vi "AlGaInPAs_v20.vi"(2 "Debug Mode":bool, 3 "Elapsed Time(s)":dbl, 4 "State":enum16{"Edit", "Start", "Run", "End", "Idle"}(ring), 5 "Argument List In":string[](array[string])) -> (0 "Status Out":string, 1 "Argument List Out":string[](array[string]))   [LabVIEW 2011]
uses:
  high_level_proc/source_noDilute.ctl
  high_level_proc/source_noDilution.ctl
panel:
  in  "Array":refnum<vi>[](array[refnum])
  in  "Al bubbler":T1 caption="Al" {"Flow" format="%.2f"}
  in  "Se bubbler":T2={"Dilution"=FALSE, "Calculated"=0, "MFC1 flow"=0.0, "MFC2 flow"=10.0, "MFC3 flow"=100.0, "Bubbler (main)"={"Flow"=0.0, "Prep"=FALSE, "Run"=FALSE, "Active"=FALSE}} caption="Al" {"Bubbler (main)"."Flow" format="%.2f"; "MFC1 flow" format="%.4f"; "MFC3 flow" format="%.1f"; "MFC2 flow" format="%.2f"; "Calculated" items=["Flow", "MFC1", "MFC2", "MFC3"]}
  in  "P bubbler":T1 caption="Al" {"Flow" format="%.2f"}
  in  "As gas":T1 caption="Al" {"Flow" format="%.2f"}
  in  "P gas":T1 caption="Al" {"Flow" format="%.2f"}
  in  "In bubbler":T1 caption="Al" {"Flow" format="%.2f"}
  in  "Tab Control":T3(tab)
  out "Al Prep":bool caption="Pre-run"
  out "Al Run":bool caption="Run"
  out "Al Flow":dbl caption="Al Flow (0-100 sscm)" format="%.2f"
  out "Ga MFC1 flow":dbl caption="R1 (0-10 sscm)" format="%.4f"
  out "Ga MFC3 flow":dbl=100.0 caption="R3 (0-1000 sscm)" format="%.1f"
  out "Ga MFC2 flow":dbl=10.0 caption="R2 (0-100 sscm)" format="%.2f"
  out "Ga Calculated":u16(ring)=1 caption="Calculated" items=["Ga flow", "MFC1", "MFC2", "MFC3"]
  out "Ga Dilution":bool caption="Dilute"
  out "Ga Prep":bool caption="Pre-run"
  out "Ga Run":bool caption="Run"
  out "Ga Flow":dbl caption="Ga Flow (0-10 sscm)" format="%.2f"
  out "In Prep":bool caption="Pre-run"
  out "In Run":bool caption="Run"
  out "In Flow":dbl caption="In Flow (0-100 sscm)" format="%.2f"
  out "P gas Run":bool caption="Run"
  out "P gas Prep":bool caption="Pre-run"
  out "P gas Flow":dbl caption="PH3 Flow (0-100 sscm)" format="%.2f"
  out "As gas Prep":bool caption="Pre-run"
  out "As gas Run":bool caption="Run"
  out "As gas Flow":dbl caption="AsH3 Flow (0-10 sscm)" format="%.2f"
  out "P liq Prep":bool caption="Pre-run"
  out "P liq Run":bool caption="Run"
  out "P liq Flow":dbl caption="P bubbler Flow (0-100 sscm)" format="%.2f"
  out "Se MFC1 flow":dbl caption="R1 (0-10 sscm)" format="%.4f"
  out "Se MFC3 flow":dbl=100.0 caption="R3 (0-1000 sscm)" format="%.1f"
  out "Se MFC2 flow":dbl=10.0 caption="R2 (0-100 sscm)" format="%.2f"
  out "Se Calculated":u16(ring)=1 caption="Calculated" items=["Ga flow", "MFC1", "MFC2", "MFC3"]
  out "Se Dilution":bool caption="Dilute"
  out "Se Prep":bool caption="Pre-run"
  out "Se Run":bool caption="Run"
  out "Se Flow":dbl caption="Se Flow (0-10 sscm)" format="%.2f"
  in  "Ga bubbler":T2={"Dilution"=FALSE, "Calculated"=0, "MFC1 flow"=0.0, "MFC2 flow"=10.0, "MFC3 flow"=100.0, "Bubbler (main)"={"Flow"=0.0, "Prep"=FALSE, "Run"=FALSE, "Active"=FALSE}} caption="Al" {"Bubbler (main)"."Flow" format="%.2f"; "MFC1 flow" format="%.4f"; "MFC3 flow" format="%.1f"; "MFC2 flow" format="%.2f"; "Calculated" items=["Flow", "MFC1", "MFC2", "MFC3"]}
  out "prep_done":bool
  out "run started":bool
  out "first":bool=TRUE
  out "total time":dbl
  out "is OK?":bool
  in  "prep_time":dbl
  in  "Cancel":bool
  in  "OK":bool
  out "tTotal(s) 2":dbl
  # "s"
  # "Add pre-run time to run time in editor."
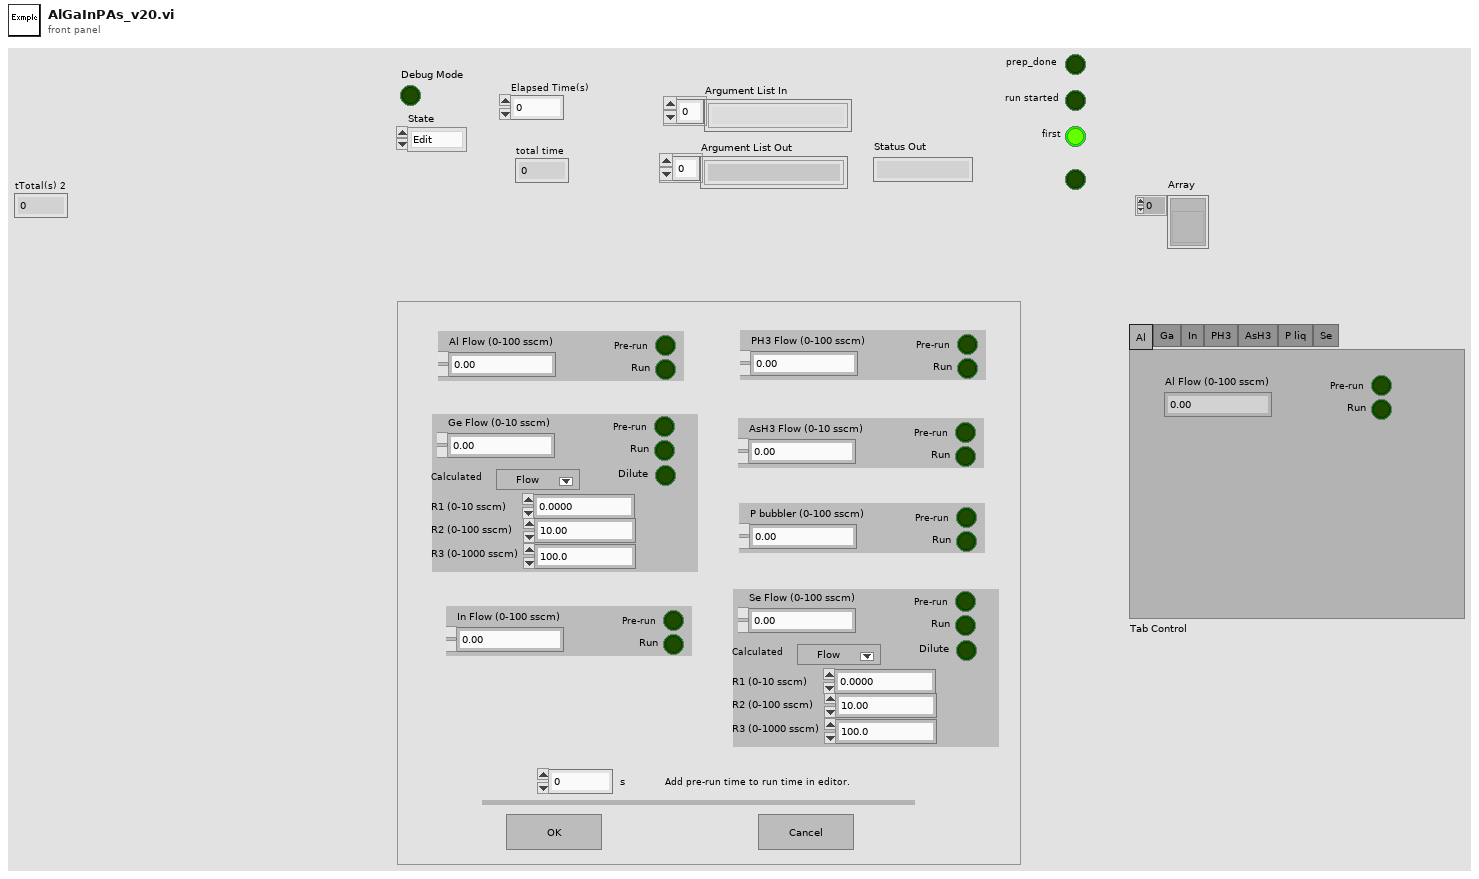
[diagram p1: front panel]
types:
  T1 = typedef "source_noDilution.ctl" = cluster{"Flow":dbl, "Prep":bool, "Run":bool, "Active":bool}
  T2 = typedef "source_noDilute.ctl" = cluster{"Dilution":bool, "Calculated":u16, "MFC1 flow":dbl, "MFC2 flow":dbl, "MFC3 flow":dbl, "Bubbler (main)":T1}
  T3 = enum32{"Al", "Ga", "In", "PH3", "AsH3", "P liq", "Se"}
  T4 = enum16{"Discrete", "Continuous", "Instantaneous", "Finite"}
  T5 = enum32{"Invalid", "Default", "Floating", "Floating/Auto-Hide", "Modal"}
  T6 = cluster{"Flow":dbl, "Prep":bool, "Run":bool, "Active":bool}
  T7 = cluster{"Dilution":bool, "Calculated":u16, "MFC1 flow":dbl, "MFC2 flow":dbl, "MFC3 flow":dbl, "Bubbler (main)":T1}
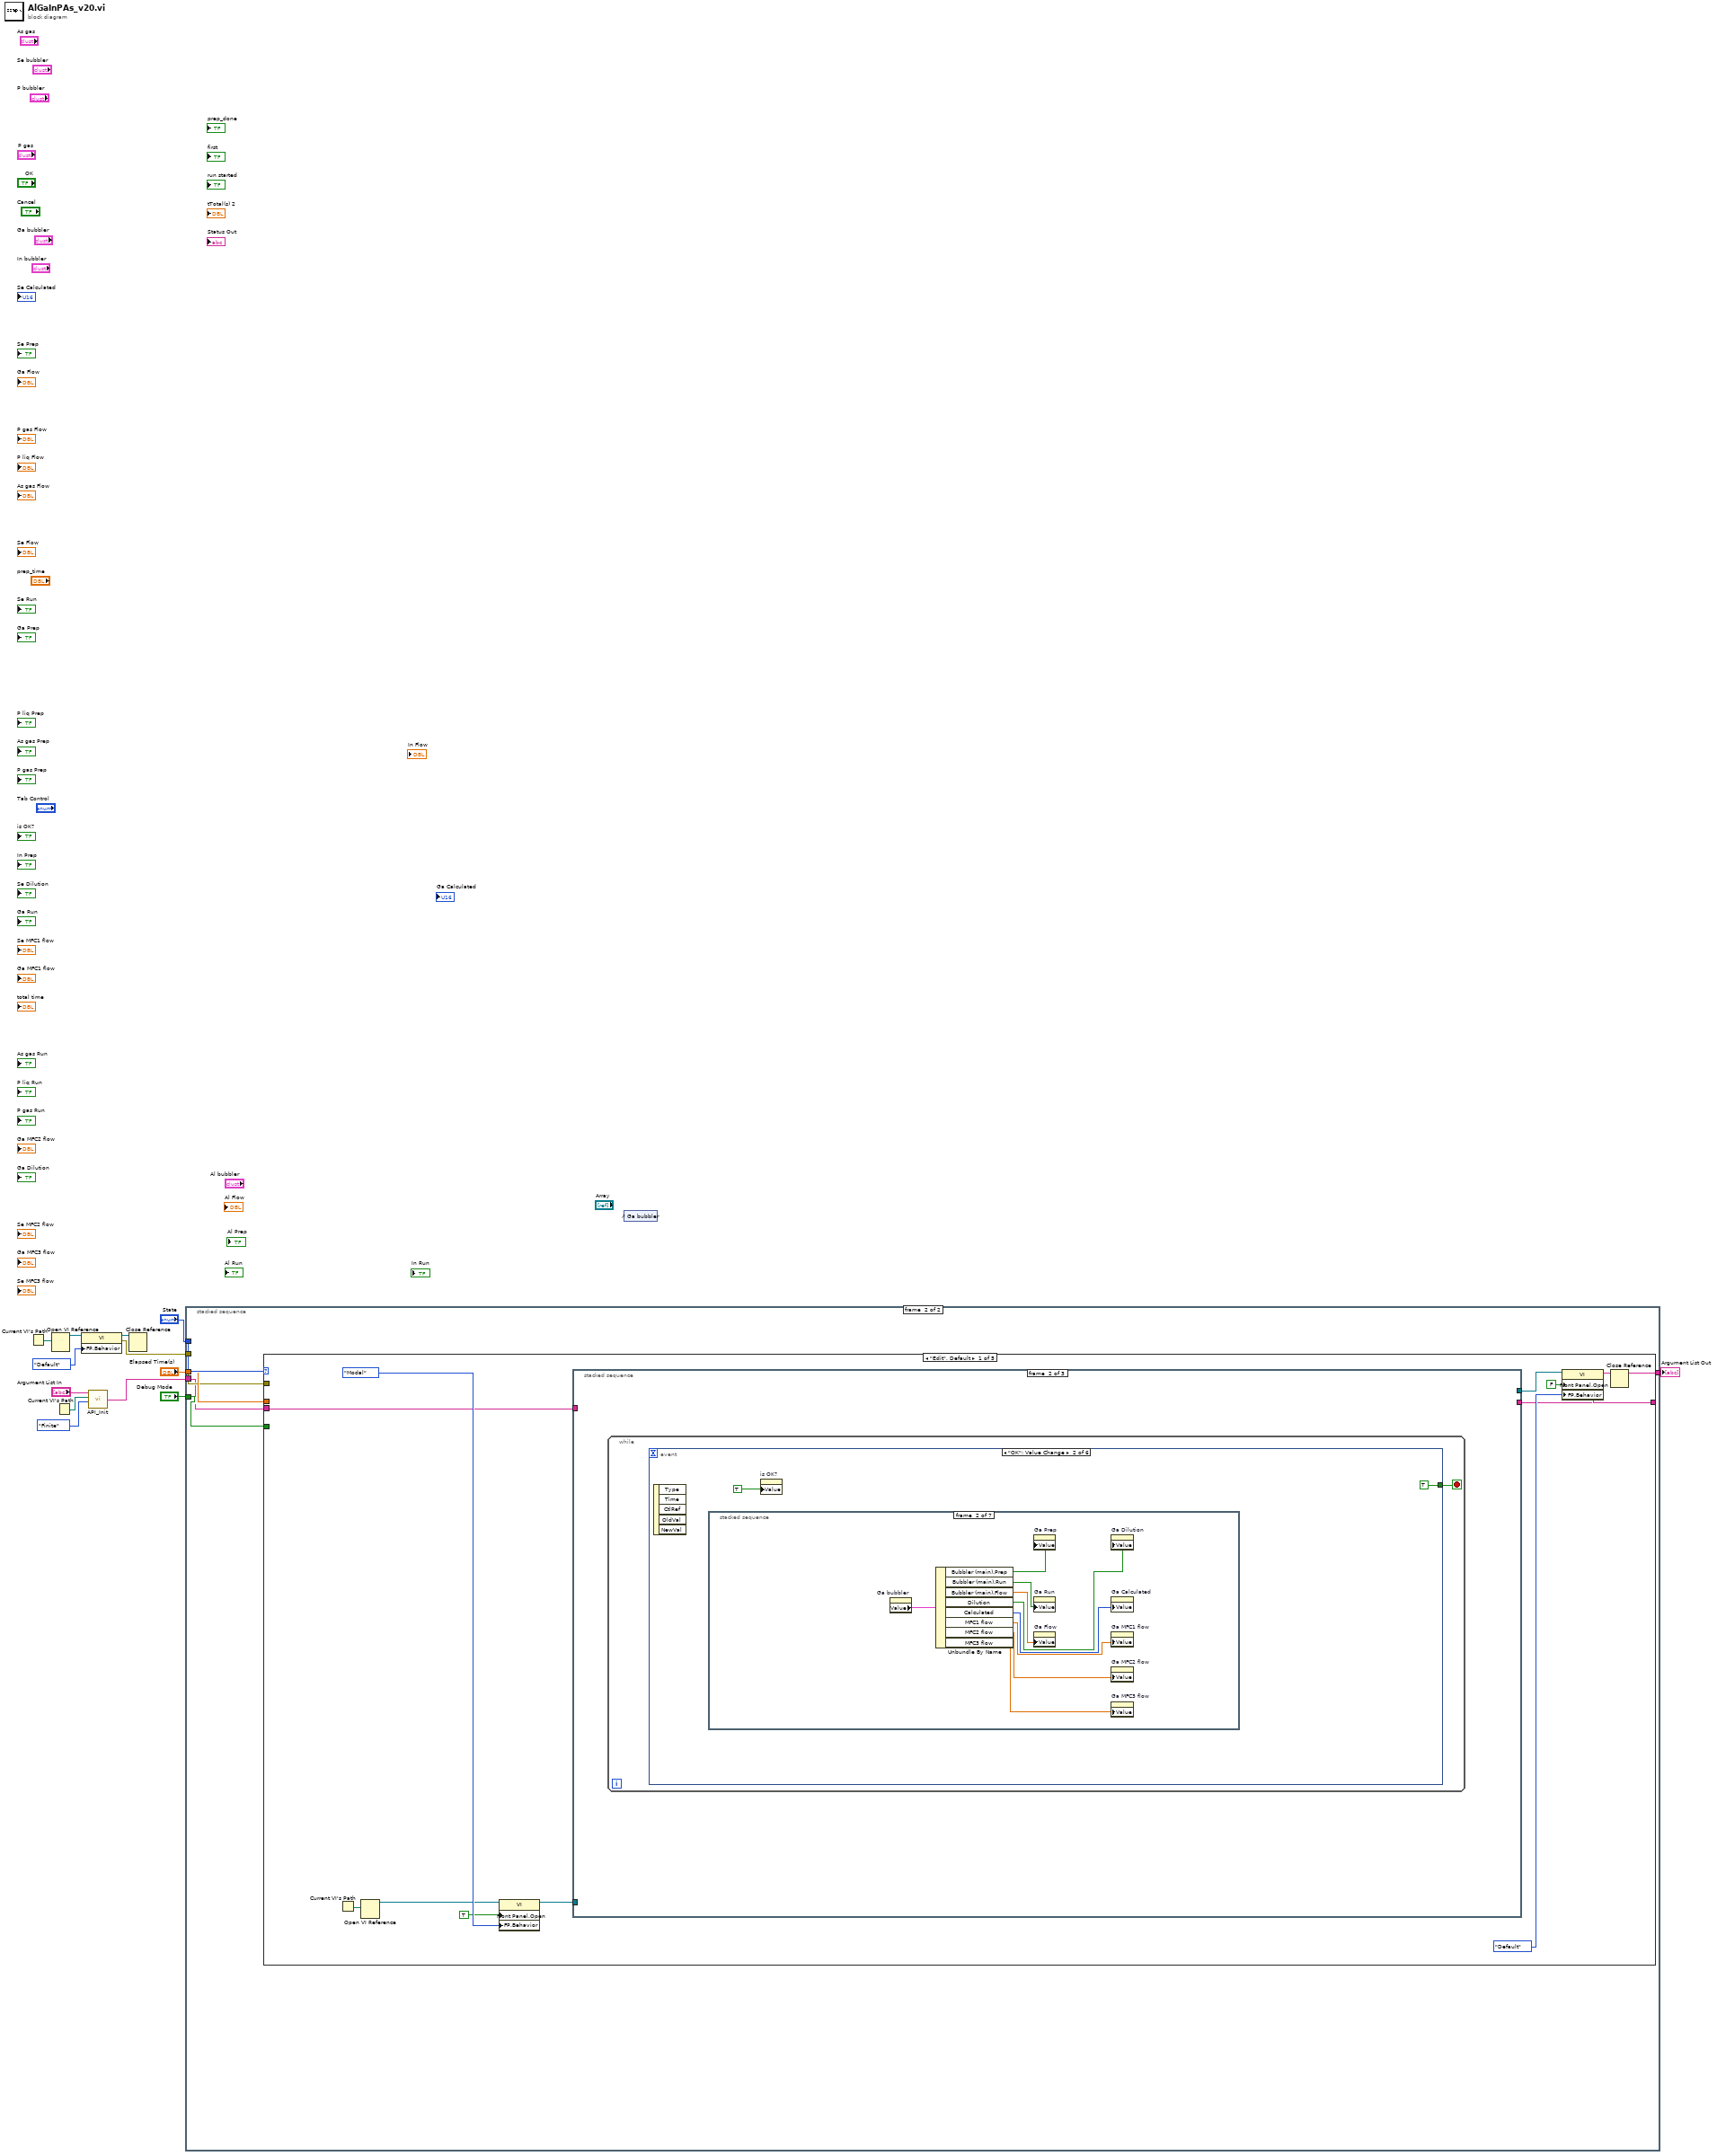
[diagram p0: block diagram]
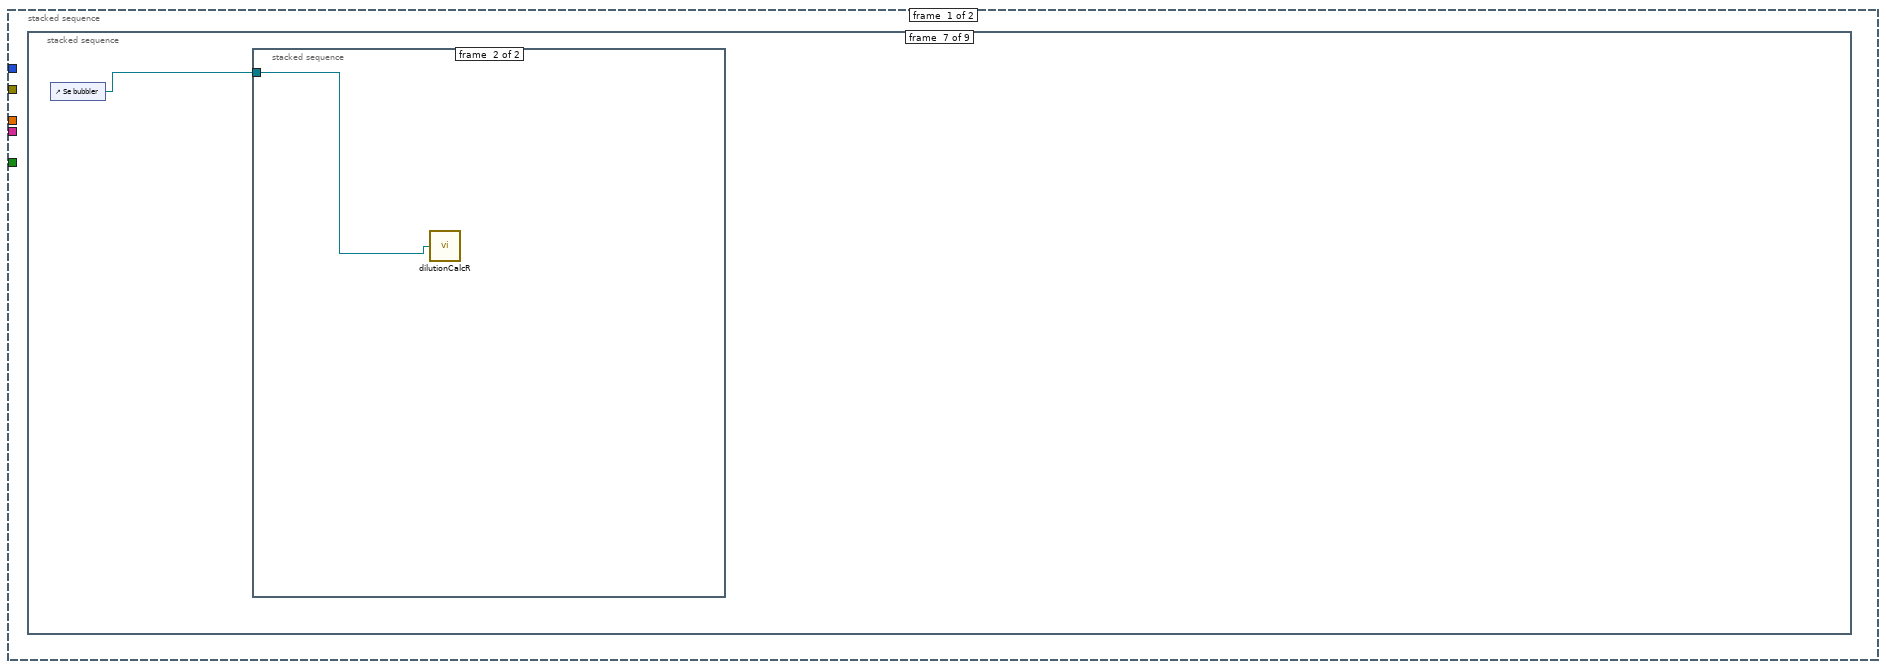
[diagram p2: hidden frame]
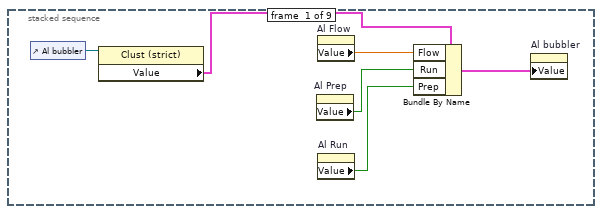
[diagram p3: hidden frame]
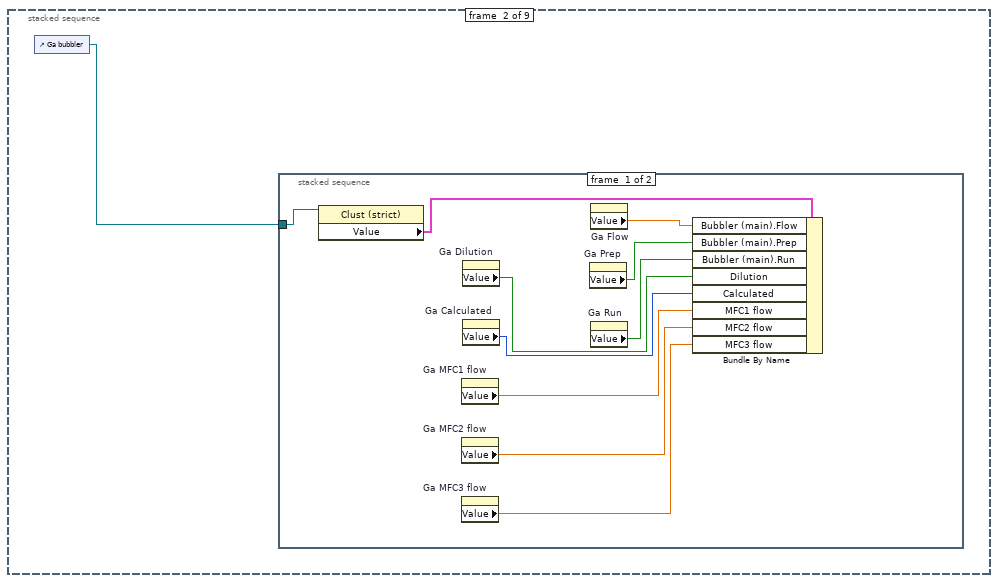
[diagram p4: hidden frame]
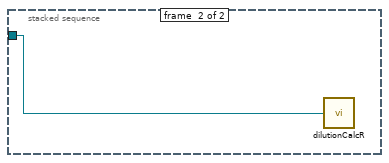
[diagram p5: hidden frame]
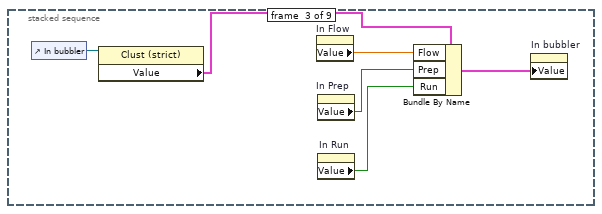
[diagram p6: hidden frame]
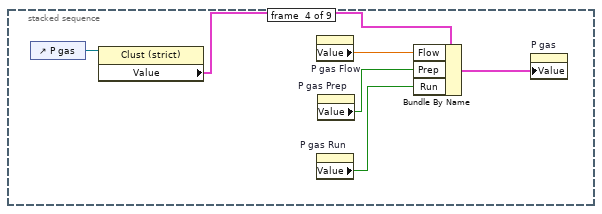
[diagram p7: hidden frame]
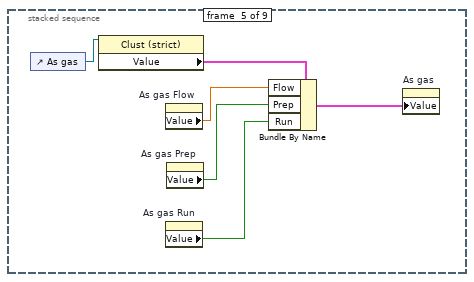
[diagram p8: hidden frame]
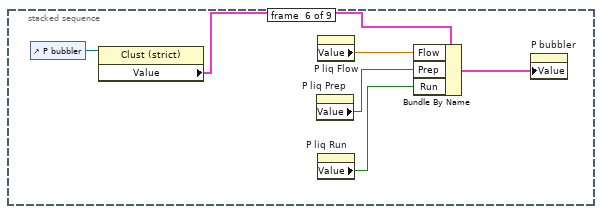
[diagram p9: hidden frame]
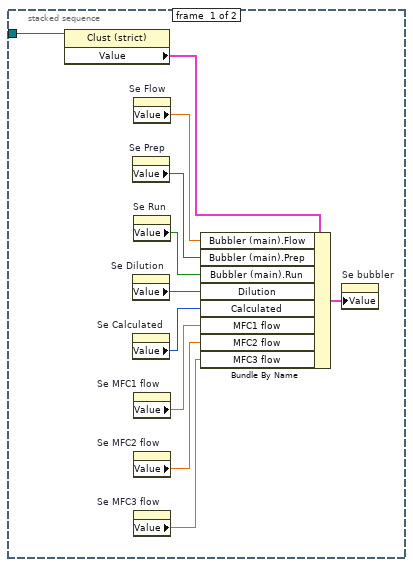
[diagram p10: hidden frame]
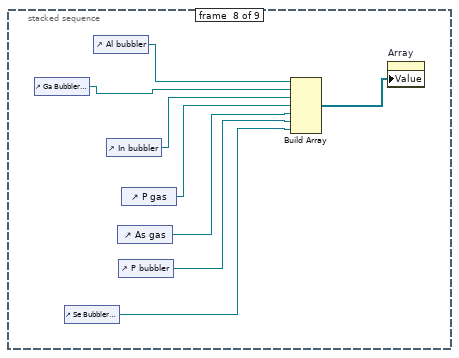
[diagram p11: hidden frame]
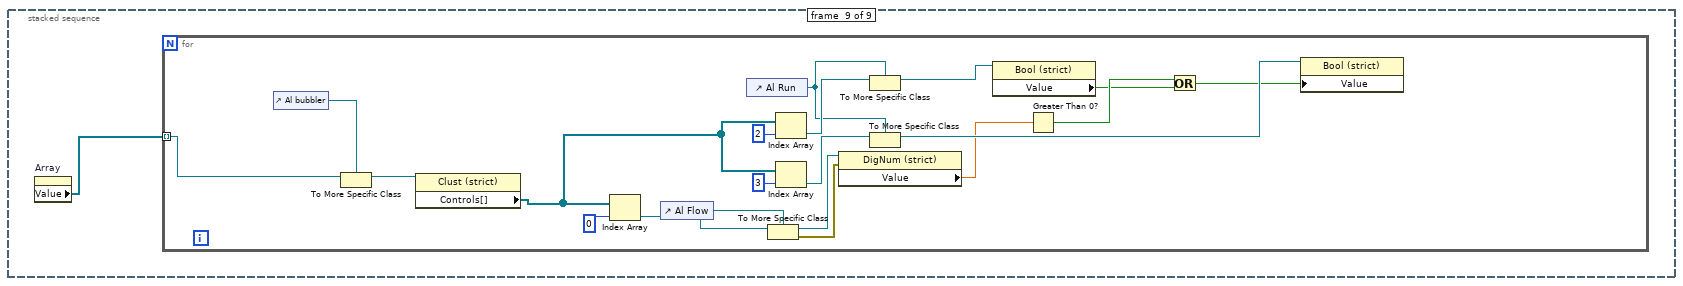
[diagram p12: hidden frame]
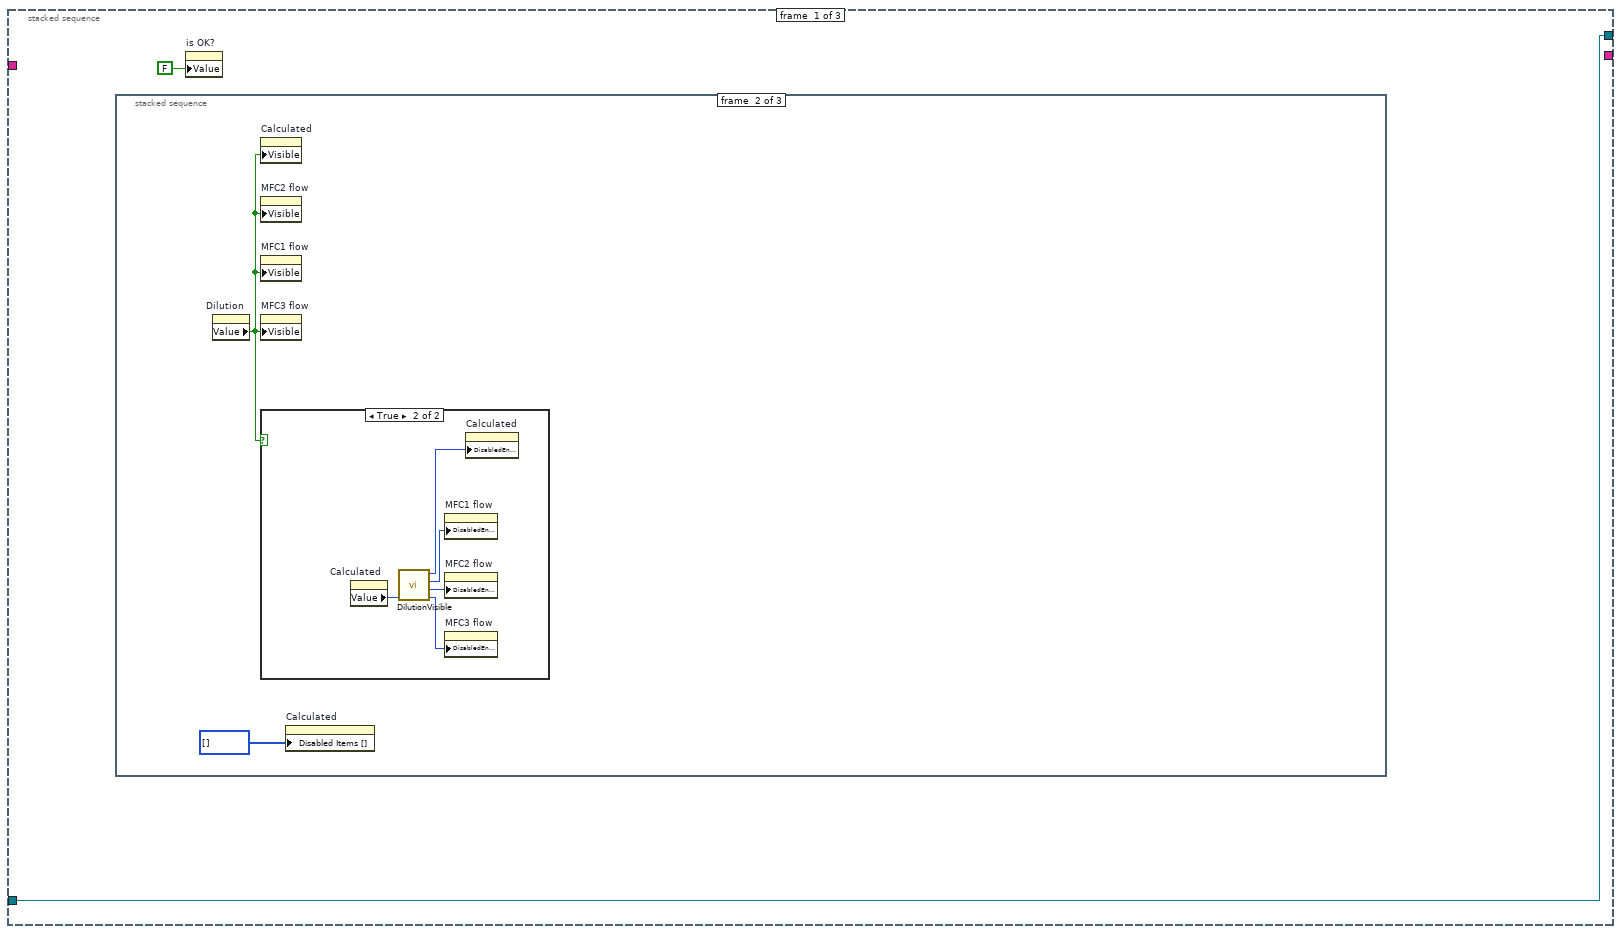
[diagram p13: hidden frame]
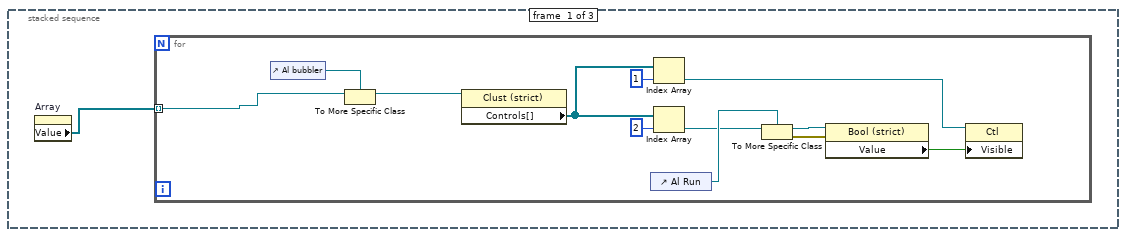
[diagram p14: hidden frame]
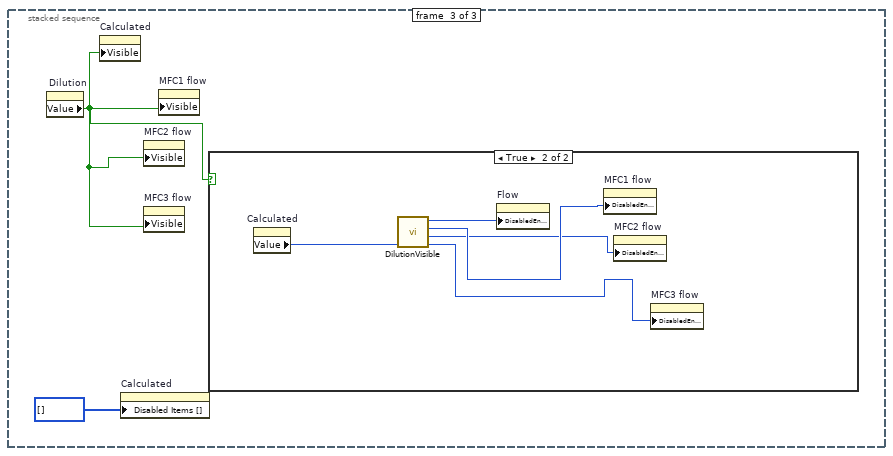
[diagram p16: hidden frame]
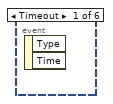
[diagram p18: hidden frame]
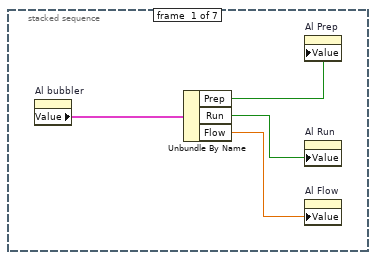
[diagram p19: hidden frame]
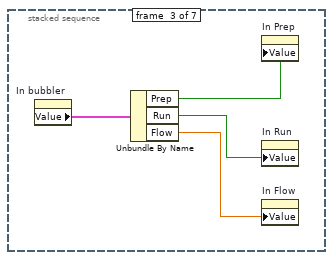
[diagram p20: hidden frame]
diagram:
  n1 = Current VI's Path() -> (path=w9:path)
  n2 = Open VI Reference(vi path=w9) -> (vi reference=w8:refnum<vi>)  [unwired: 1 in, 5 out]
  n3 = Current VI's Path() -> (path=w4:path)
  n4 = property class="VI"(reference=w8, "FP.Behavior"=T5."Default" ("Front Panel Window:Behavior")) -> (reference out=w6:refnum<vi>, error out=w5:errorcluster)  [unwired: 1 in]
  n5 = call "API_Init.vi"("API Mode"=T4."Finite", "VI Path"=w4, "Argument List In"="Argument List In") -> ("Argument List Out"=w1:string[])  [unwired: 1 in]
  n6 = Close Reference(reference=w6) -> ()  [unwired: 1 in, 1 out]
  n7 = stacked-sequence {
    tunnel: "State" -> [_ w103]
    tunnel: "Debug Mode" -> [_ w102]
    tunnel: "Elapsed Time(s)" -> [_ w101]
    tunnel: [_ w100] -> w10
    tunnel: w5 -> [_ w99]
    tunnel: w1 -> [_ w98]
    frame #0 {
      n8 = stacked-sequence {
        frame #0 {
          n9 = control-ref of="Al bubbler"() -> (w16:refnum<vi>)
          n10 = property class="Clust (strict)"(reference=w16) -> ("Value"=w15:T6)  [unwired: 1 in, 2 out]
          n11 = property on="Al Prep" class="Bool (strict)"() -> ("Value"=w18:bool)  [unwired: 2 in, 2 out]
          n12 = property on="Al Flow" class="DigNum (strict)"() -> ("Value"=w19:dbl)  [unwired: 2 in, 2 out]
          n13 = property on="Al Run" class="Bool (strict)"() -> ("Value"=w17:bool)  [unwired: 2 in, 2 out]
          n14 = Bundle By Name(cluster=w15, "Flow"=w19, "Run"=w18, "Prep"=w17) -> (w14:T6)
          n15 = property on="Al bubbler" class="Clust (strict)"("Value"=w14) -> ()  [unwired: 2 in, 2 out]
        }
        frame #1 {
          n16 = control-ref of="Ga bubbler"() -> (w20:refnum<vi>)
          n17 = stacked-sequence {
            tunnel: w20 -> [w22 w31]
            frame #0 {
              n18 = property class="Clust (strict)"(reference=w22) -> ("Value"=w21:T7)  [unwired: 1 in, 2 out]
              n19 = property on="Ga MFC1 flow" class="DigNum (strict)"() -> ("Value"=w28:dbl)  [unwired: 2 in, 2 out]
              n20 = property on="Ga MFC2 flow" class="DigNum (strict)"() -> ("Value"=w29:dbl)  [unwired: 2 in, 2 out]
              n21 = property on="Ga MFC3 flow" class="DigNum (strict)"() -> ("Value"=w30:dbl)  [unwired: 2 in, 2 out]
              n22 = property on="Ga Dilution" class="Bool (strict)"() -> ("Value"=w27:bool)  [unwired: 2 in, 2 out]
              n23 = property on="Ga Calculated" class="Ring (strict)"() -> ("Value"=w25:u16)  [unwired: 2 in, 2 out]
              n24 = property on="Ga Prep" class="Bool (strict)"() -> ("Value"=w24:bool)  [unwired: 2 in, 2 out]
              n25 = property on="Ga Flow" class="DigNum (strict)"() -> ("Value"=w23:dbl)  [unwired: 2 in, 2 out]
              n26 = property on="Ga Run" class="Bool (strict)"() -> ("Value"=w26:bool)  [unwired: 2 in, 2 out]
              n27 = Bundle By Name(cluster=w21, "Bubbler (main).Flow"=w23, "Bubbler (main).Prep"=w24, "Bubbler (main).Run"=w26, "Dilution"=w27, "Calculated"=w25, "MFC1 flow"=w28, "MFC2 flow"=w29, "MFC3 flow"=w30) -> ()  [unwired: 1 out]
            }
            frame #1 {
              n28 = call "dilutionCalcR.vi"("Clust Refnum"=w31) -> ()
            }
          }
        }
        frame #2 {
          n29 = control-ref of="In bubbler"() -> (w32:refnum<vi>)
          n30 = property class="Clust (strict)"(reference=w32) -> ("Value"=w33:T6)  [unwired: 1 in, 2 out]
          n31 = property on="In Flow" class="DigNum (strict)"() -> ("Value"=w34:dbl)  [unwired: 2 in, 2 out]
          n32 = property on="In Prep" class="Bool (strict)"() -> ("Value"=w36:bool)  [unwired: 2 in, 2 out]
          n33 = property on="In Run" class="Bool (strict)"() -> ("Value"=w37:bool)  [unwired: 2 in, 2 out]
          n34 = Bundle By Name(cluster=w33, "Flow"=w34, "Prep"=w36, "Run"=w37) -> (w35:T6)
          n35 = property on="In bubbler" class="Clust (strict)"("Value"=w35) -> ()  [unwired: 2 in, 2 out]
        }
        frame #3 {
          n36 = control-ref of="P gas"() -> (w38:refnum<vi>)
          n37 = property class="Clust (strict)"(reference=w38) -> ("Value"=w39:T6)  [unwired: 1 in, 2 out]
          n38 = property on="P gas Flow" class="DigNum (strict)"() -> ("Value"=w40:dbl)  [unwired: 2 in, 2 out]
          n39 = property on="P gas Run" class="Bool (strict)"() -> ("Value"=w43:bool)  [unwired: 2 in, 2 out]
          n40 = property on="P gas Prep" class="Bool (strict)"() -> ("Value"=w42:bool)  [unwired: 2 in, 2 out]
          n41 = Bundle By Name(cluster=w39, "Flow"=w40, "Prep"=w42, "Run"=w43) -> (w41:T6)
          n42 = property on="P gas" class="Clust (strict)"("Value"=w41) -> ()  [unwired: 2 in, 2 out]
        }
        frame #4 {
          n43 = control-ref of="As gas"() -> (w45:refnum<vi>)
          n44 = property class="Clust (strict)"(reference=w45) -> ("Value"=w44:T6)  [unwired: 1 in, 2 out]
          n45 = property on="As gas Flow" class="DigNum (strict)"() -> ("Value"=w47:dbl)  [unwired: 2 in, 2 out]
          n46 = property on="As gas Run" class="Bool (strict)"() -> ("Value"=w49:bool)  [unwired: 2 in, 2 out]
          n47 = property on="As gas Prep" class="Bool (strict)"() -> ("Value"=w48:bool)  [unwired: 2 in, 2 out]
          n48 = Bundle By Name(cluster=w44, "Flow"=w47, "Prep"=w48, "Run"=w49) -> (w46:T6)
          n49 = property on="As gas" class="Clust (strict)"("Value"=w46) -> ()  [unwired: 2 in, 2 out]
        }
        frame #5 {
          n50 = control-ref of="P bubbler"() -> (w50:refnum<vi>)
          n51 = property class="Clust (strict)"(reference=w50) -> ("Value"=w51:T6)  [unwired: 1 in, 2 out]
          n52 = property on="P liq Prep" class="Bool (strict)"() -> ("Value"=w54:bool)  [unwired: 2 in, 2 out]
          n53 = property on="P liq Flow" class="DigNum (strict)"() -> ("Value"=w53:dbl)  [unwired: 2 in, 2 out]
          n54 = property on="P liq Run" class="Bool (strict)"() -> ("Value"=w55:bool)  [unwired: 2 in, 2 out]
          n55 = Bundle By Name(cluster=w51, "Flow"=w53, "Prep"=w54, "Run"=w55) -> (w52:T6)
          n56 = property on="P bubbler" class="Clust (strict)"("Value"=w52) -> ()  [unwired: 2 in, 2 out]
        }
        frame #6 {
          n57 = control-ref of="Se bubbler"() -> (w56:refnum<vi>)
          n58 = stacked-sequence {
            tunnel: w56 -> [w57 w68]
            frame #0 {
              n59 = property class="Clust (strict)"(reference=w57) -> ("Value"=w58:T7)  [unwired: 1 in, 2 out]
              n60 = property on="Se Prep" class="Bool (strict)"() -> ("Value"=w61:bool)  [unwired: 2 in, 2 out]
              n61 = property on="Se Dilution" class="Bool (strict)"() -> ("Value"=w63:bool)  [unwired: 2 in, 2 out]
              n62 = property on="Se Calculated" class="Ring (strict)"() -> ("Value"=w64:u16)  [unwired: 2 in, 2 out]
              n63 = property on="Se Flow" class="DigNum (strict)"() -> ("Value"=w60:dbl)  [unwired: 2 in, 2 out]
              n64 = property on="Se Run" class="Bool (strict)"() -> ("Value"=w62:bool)  [unwired: 2 in, 2 out]
              n65 = property on="Se MFC1 flow" class="DigNum (strict)"() -> ("Value"=w65:dbl)  [unwired: 2 in, 2 out]
              n66 = property on="Se MFC2 flow" class="DigNum (strict)"() -> ("Value"=w66:dbl)  [unwired: 2 in, 2 out]
              n67 = property on="Se MFC3 flow" class="DigNum (strict)"() -> ("Value"=w67:dbl)  [unwired: 2 in, 2 out]
              n68 = Bundle By Name(cluster=w58, "Bubbler (main).Flow"=w60, "Bubbler (main).Prep"=w61, "Bubbler (main).Run"=w62, "Dilution"=w63, "Calculated"=w64, "MFC1 flow"=w65, "MFC2 flow"=w66, "MFC3 flow"=w67) -> (w59:T7)
              n69 = property on="Se bubbler" class="Clust (strict)"("Value"=w59) -> ()  [unwired: 2 in, 2 out]
            }
            frame #1 {
              n70 = call "dilutionCalcR.vi"("Clust Refnum"=w68) -> ()
            }
          }
        }
        frame #7 {
          n71 = control-ref of="Ga Bubbler (main)"() -> (w70:refnum<vi>)
          n72 = control-ref of="Se Bubbler (main)"() -> (w69:refnum<vi>)
          n73 = control-ref of="Al bubbler"() -> (w75:refnum<vi>)
          n74 = control-ref of="In bubbler"() -> (w74:refnum<vi>)
          n75 = control-ref of="As gas"() -> (w72:refnum<vi>)
          n76 = control-ref of="P bubbler"() -> (w71:refnum<vi>)
          n77 = control-ref of="P gas"() -> (w73:refnum<vi>)
          n78 = Build Array(w75, w70, w74, w73, w72, w71, w69) -> (w76:refnum<vi>[])
          n79 = property on="Array" class="Arr (strict)"("Value"=w76) -> ()  [unwired: 2 in, 2 out]
        }
        frame #8 {
          n80 = property on="Array" class="Arr (strict)"() -> ("Value"=w77:refnum<vi>[])  [unwired: 2 in, 2 out]
          n81 = for {
            tunnel: w77 -> [w78] mode=indexing
            n82 = control-ref of="Al bubbler"() -> (w81:refnum<vi>)
            n83 = To More Specific Class(target class=w81, reference=w78) -> (specific class reference=w80:refnum<vi>)  [unwired: 1 in, 1 out]
            n84 = property class="Clust (strict)"(reference=w80) -> ("Controls[]"=w79:refnum<vi>[])  [unwired: 1 in, 2 out]
            n85 = Index Array(array=w79, index=0) -> (element=w93:refnum<vi>)
            n86 = control-ref of="Al Flow"() -> (w92:refnum<vi>)
            n87 = control-ref of="Al Run"() -> (w94:refnum<vi>)
            n88 = To More Specific Class(target class=w92, reference=w93) -> (specific class reference=w89:refnum<vi>, error out=w88:errorcluster)  [unwired: 1 in]
            n89 = Index Array(array=w79, index=2) -> (element=w96:refnum<vi>)
            n90 = Index Array(array=w79, index=3) -> (element=w95:refnum<vi>)
            n91 = property class="DigNum (strict)"(reference=w89, error in=w88) -> ("Value"=w87:dbl)  [unwired: 2 out]
            n92 = To More Specific Class(target class=w94, reference=w96) -> (specific class reference=w91:refnum<vi>)  [unwired: 1 in, 1 out]
            n93 = To More Specific Class(target class=w94, reference=w95) -> (specific class reference=w90:refnum<vi>)  [unwired: 1 in, 1 out]
            n94 = property class="Bool (strict)"(reference=w91) -> ("Value"=w86:bool)  [unwired: 1 in, 2 out]
            n95 = Greater Than 0?(x=w87) -> (x > 0?=w97:bool)
            n96 = Or(x=w97, y=w86) -> (x .or. y?=w85:bool)
            n97 = property class="Bool (strict)"(reference=w90, "Value"=w85) -> ()  [unwired: 1 in, 2 out]
          }
        }
      }
    }
    frame #1 {
      n98 = case shown="\"Edit\", Default" w103 {
        tunnel: w102 -> [_ w207 w225 _ _]
        tunnel: w101 -> [_ _ w226 _ _]
        tunnel: w98 -> [w105 w212 w224 w328 w329]
        tunnel: [w104 w211 w223 w328 w329] -> w100
        tunnel: w99 -> [_ _ _ _ _]
        frame "Edit", Default {
          n99 = Current VI's Path() -> (path=w110:path)
          n100 = Open VI Reference(vi path=w110) -> (vi reference=w109:refnum<vi>)  [unwired: 1 in, 5 out]
          n101 = property class="VI"(reference=w109, "Front Panel.Open"=TRUE ("Front Panel Window:Open"), "FP.Behavior"=T5."Modal" ("Front Panel Window:Behavior")) -> (reference out=w108:refnum<vi>)  [unwired: 1 in, 1 out]
          n102 = stacked-sequence {
            tunnel: w105 -> [_ _ w202]
            tunnel: w108 -> [w116 _ _]
            tunnel: [w116 _ _] -> w112
            tunnel: [_ _ w203] -> w104
            frame #0 {
              n103 = stacked-sequence {
                frame #0 {
                  n104 = property on="Array" class="Arr (strict)"() -> ("Value"=w117:refnum<vi>[])  [unwired: 2 in, 2 out]
                  n105 = for {
                    tunnel: w117 -> [w118] mode=indexing
                    n106 = control-ref of="Al bubbler"() -> (w119:refnum<vi>)
                    n107 = To More Specific Class(target class=w119, reference=w118) -> (specific class reference=w127:refnum<vi>)  [unwired: 1 in, 1 out]
                    n108 = property class="Clust (strict)"(reference=w127) -> ("Controls[]"=w126:refnum<vi>[])  [unwired: 1 in, 2 out]
                    n109 = control-ref of="Al Run"() -> (w124:refnum<vi>)
                    n110 = Index Array(array=w126, index=1) -> (element=w128:refnum<vi>)
                    n111 = Index Array(array=w126, index=2) -> (element=w123:refnum<vi>)
                    n112 = To More Specific Class(target class=w124, reference=w123) -> (specific class reference=w122:refnum<vi>, error out=w121:errorcluster)  [unwired: 1 in]
                    n113 = property class="Bool (strict)"(reference=w122, error in=w121) -> ("Value"=w120:bool)  [unwired: 2 out]
                    n114 = property class="Ctl"(reference=w128, "Visible"=w120) -> ()  [unwired: 1 in, 2 out]
                  }
                }
                frame #1 {
                  n115 = property on="Dilution" class="Bool (strict)"() -> ("Value"=w131:bool)  [unwired: 2 in, 2 out]
                  n116 = property on="Calculated" class="Ring (strict)"("Visible"=w131) -> ()  [unwired: 2 in, 2 out]
                  n117 = property on="MFC2 flow" class="DigNum (strict)"("Visible"=w131) -> ()  [unwired: 2 in, 2 out]
                  n118 = property on="MFC1 flow" class="DigNum (strict)"("Visible"=w131) -> ()  [unwired: 2 in, 2 out]
                  n119 = property on="MFC3 flow" class="DigNum (strict)"("Visible"=w131) -> ()  [unwired: 2 in, 2 out]
                  n120 = case shown="True" w131 {
                    frame False {
                    }
                    frame True {
                      n121 = property on="Calculated" class="Ring (strict)"() -> ("Value"=w133:u16)  [unwired: 2 in, 2 out]
                      n122 = call "DilutionVisible.vi"("calculated"=w133) -> ("MFC3"=w136:u16, "MFC2"=w135:u16, "MFC1"=w134:u16, "flow"=w132:u16)  [unwired: 3 in]
                      n123 = property on="MFC1 flow" class="DigNum (strict)"("DisabledEnum"=w134) -> ()  [unwired: 2 in, 2 out]
                      n124 = property on="MFC2 flow" class="DigNum (strict)"("DisabledEnum"=w135) -> ()  [unwired: 2 in, 2 out]
                      n125 = property on="MFC3 flow" class="DigNum (strict)"("DisabledEnum"=w136) -> ()  [unwired: 2 in, 2 out]
                      n126 = property on="Calculated" class="Ring (strict)"("DisabledEnum"=w132) -> ()  [unwired: 2 in, 2 out]
                    }
                  }
                  n127 = property on="Calculated" class="Ring (strict)"("Disabled Items []"=i32[] []) -> ()  [unwired: 2 in, 2 out]
                }
                frame #2 {
                  n128 = property on="Dilution" class="Bool (strict)"() -> ("Value"=w137:bool)  [unwired: 2 in, 2 out]
                  n129 = property on="Calculated" class="Ring (strict)"("Visible"=w137) -> ()  [unwired: 2 in, 2 out]
                  n130 = property on="Calculated" class="Ring (strict)"("Disabled Items []"=i32[] []) -> ()  [unwired: 2 in, 2 out]
                  n131 = property on="MFC2 flow" class="DigNum (strict)"("Visible"=w137) -> ()  [unwired: 2 in, 2 out]
                  n132 = property on="MFC3 flow" class="DigNum (strict)"("Visible"=w137) -> ()  [unwired: 2 in, 2 out]
                  n133 = property on="MFC1 flow" class="DigNum (strict)"("Visible"=w137) -> ()  [unwired: 2 in, 2 out]
                  n134 = case shown="True" w137 {
                    frame False {
                    }
                    frame True {
                      n135 = property on="Calculated" class="Ring (strict)"() -> ("Value"=w142:u16)  [unwired: 2 in, 2 out]
                      n136 = call "DilutionVisible.vi"("calculated"=w142) -> ("MFC3"=w140:u16, "MFC2"=w139:u16, "MFC1"=w141:u16, "flow"=w143:u16)  [unwired: 3 in]
                      n137 = property on="Flow" class="DigNum (strict)"("DisabledEnum"=w143) -> ()  [unwired: 2 in, 2 out]
                      n138 = property on="MFC1 flow" class="DigNum (strict)"("DisabledEnum"=w141) -> ()  [unwired: 2 in, 2 out]
                      n139 = property on="MFC2 flow" class="DigNum (strict)"("DisabledEnum"=w139) -> ()  [unwired: 2 in, 2 out]
                      n140 = property on="MFC3 flow" class="DigNum (strict)"("DisabledEnum"=w140) -> ()  [unwired: 2 in, 2 out]
                    }
                  }
                }
              }
              n141 = property on="is OK?" class="Bool (strict)"("Value"=FALSE ("is OK?")) -> ()  [unwired: 2 in, 2 out]
            }
            frame #1 {
              n142 = while {
                stop <- w144 stop-if-true
                n143 = event shown="[1] \"OK\": Value Change" {
                  selector: _ -> [_ _ _ _ _ _]
                  dyn-events: _ -> [_ _ _ _ _ _]
                  timeout: _ -> [_ _ _ _ _ _]
                  tunnel: [_ TRUE _ TRUE _ _] -> w144
                  event Timeout {
                    n144 = event-data() -> ()  [unwired: 1 in, 2 out]
                  }
                  event "OK": Value Change {
                    n145 = event-data() -> ()  [unwired: 1 in, 5 out]
                    n146 = stacked-sequence {
                      frame #0 {
                        n147 = property on="Al bubbler" class="Clust (strict)"() -> ("Value"=w147:T6)  [unwired: 2 in, 2 out]
                        n148 = Unbundle By Name(w147) -> ("Prep"=w150:bool, "Run"=w149:bool, "Flow"=w148:dbl)
                        n149 = property on="Al Prep" class="Bool (strict)"("Value"=w150) -> ()  [unwired: 2 in, 2 out]
                        n150 = property on="Al Run" class="Bool (strict)"("Value"=w149) -> ()  [unwired: 2 in, 2 out]
                        n151 = property on="Al Flow" class="DigNum (strict)"("Value"=w148) -> ()  [unwired: 2 in, 2 out]
                      }
                      frame #1 {
                        n152 = property on="Ga bubbler" class="Clust (strict)"() -> ("Value"=w159:T7)  [unwired: 2 in, 2 out]
                        n153 = Unbundle By Name(w159) -> ("Bubbler (main).Prep"=w158:bool, "Bubbler (main).Run"=w157:bool, "Bubbler (main).Flow"=w156:dbl, "Dilution"=w155:bool, "Calculated"=w154:u16, "MFC1 flow"=w153:dbl, "MFC2 flow"=w152:dbl, "MFC3 flow"=w151:dbl)
                        n154 = property on="Ga Prep" class="Bool (strict)"("Value"=w158) -> ()  [unwired: 2 in, 2 out]
                        n155 = property on="Ga Run" class="Bool (strict)"("Value"=w157) -> ()  [unwired: 2 in, 2 out]
                        n156 = property on="Ga Flow" class="DigNum (strict)"("Value"=w156) -> ()  [unwired: 2 in, 2 out]
                        n157 = property on="Ga Dilution" class="Bool (strict)"("Value"=w155) -> ()  [unwired: 2 in, 2 out]
                        n158 = property on="Ga Calculated" class="Ring (strict)"("Value"=w154) -> ()  [unwired: 2 in, 2 out]
                        n159 = property on="Ga MFC1 flow" class="DigNum (strict)"("Value"=w153) -> ()  [unwired: 2 in, 2 out]
                        n160 = property on="Ga MFC2 flow" class="DigNum (strict)"("Value"=w152) -> ()  [unwired: 2 in, 2 out]
                        n161 = property on="Ga MFC3 flow" class="DigNum (strict)"("Value"=w151) -> ()  [unwired: 2 in, 2 out]
                      }
                      frame #2 {
                        n162 = property on="In bubbler" class="Clust (strict)"() -> ("Value"=w163:T6)  [unwired: 2 in, 2 out]
                        n163 = Unbundle By Name(w163) -> ("Prep"=w162:bool, "Run"=w161:bool, "Flow"=w160:dbl)
                        n164 = property on="In Prep" class="Bool (strict)"("Value"=w162) -> ()  [unwired: 2 in, 2 out]
                        n165 = property on="In Run" class="Bool (strict)"("Value"=w161) -> ()  [unwired: 2 in, 2 out]
                        n166 = property on="In Flow" class="DigNum (strict)"("Value"=w160) -> ()  [unwired: 2 in, 2 out]
                      }
                      frame #3 {
                        n167 = property on="P gas" class="Clust (strict)"() -> ("Value"=w167:T6)  [unwired: 2 in, 2 out]
                        n168 = Unbundle By Name(w167) -> ("Prep"=w166:bool, "Run"=w165:bool, "Flow"=w164:dbl)
                        n169 = property on="P gas Prep" class="Bool (strict)"("Value"=w166) -> ()  [unwired: 2 in, 2 out]
                        n170 = property on="P gas Run" class="Bool (strict)"("Value"=w165) -> ()  [unwired: 2 in, 2 out]
                        n171 = property on="P gas Flow" class="DigNum (strict)"("Value"=w164) -> ()  [unwired: 2 in, 2 out]
                      }
                      frame #4 {
                        n172 = property on="As gas" class="Clust (strict)"() -> ("Value"=w171:T6)  [unwired: 2 in, 2 out]
                        n173 = Unbundle By Name(w171) -> ("Prep"=w170:bool, "Run"=w169:bool, "Flow"=w168:dbl)
                        n174 = property on="As gas Prep" class="Bool (strict)"("Value"=w170) -> ()  [unwired: 2 in, 2 out]
                        n175 = property on="As gas Run" class="Bool (strict)"("Value"=w169) -> ()  [unwired: 2 in, 2 out]
                        n176 = property on="As gas Flow" class="DigNum (strict)"("Value"=w168) -> ()  [unwired: 2 in, 2 out]
                      }
                      frame #5 {
                        n177 = property on="P bubbler" class="Clust (strict)"() -> ("Value"=w175:T6)  [unwired: 2 in, 2 out]
                        n178 = Unbundle By Name(w175) -> ("Prep"=w174:bool, "Run"=w173:bool, "Flow"=w172:dbl)
                        n179 = property on="P liq Prep" class="Bool (strict)"("Value"=w174) -> ()  [unwired: 2 in, 2 out]
                        n180 = property on="P liq Run" class="Bool (strict)"("Value"=w173) -> ()  [unwired: 2 in, 2 out]
                        n181 = property on="P liq Flow" class="DigNum (strict)"("Value"=w172) -> ()  [unwired: 2 in, 2 out]
                      }
                      frame #6 {
                        n182 = property on="Se bubbler" class="Clust (strict)"() -> ("Value"=w184:T7)  [unwired: 2 in, 2 out]
                        n183 = Unbundle By Name(w184) -> ("Bubbler (main).Prep"=w183:bool, "Bubbler (main).Run"=w182:bool, "Bubbler (main).Flow"=w181:dbl, "Dilution"=w180:bool, "Calculated"=w179:u16, "MFC1 flow"=w178:dbl, "MFC2 flow"=w177:dbl, "MFC3 flow"=w176:dbl)
                        n184 = property on="Se Prep" class="Bool (strict)"("Value"=w183) -> ()  [unwired: 2 in, 2 out]
                        n185 = property on="Se Run" class="Bool (strict)"("Value"=w182) -> ()  [unwired: 2 in, 2 out]
                        n186 = property on="Se Flow" class="DigNum (strict)"("Value"=w181) -> ()  [unwired: 2 in, 2 out]
                        n187 = property on="Se Dilution" class="Bool (strict)"("Value"=w180) -> ()  [unwired: 2 in, 2 out]
                        n188 = property on="Se Calculated" class="Ring (strict)"("Value"=w179) -> ()  [unwired: 2 in, 2 out]
                        n189 = property on="Se MFC1 flow" class="DigNum (strict)"("Value"=w178) -> ()  [unwired: 2 in, 2 out]
                        n190 = property on="Se MFC2 flow" class="DigNum (strict)"("Value"=w177) -> ()  [unwired: 2 in, 2 out]
                        n191 = property on="Se MFC3 flow" class="DigNum (strict)"("Value"=w176) -> ()  [unwired: 2 in, 2 out]
                      }
                    }
                    n192 = property on="is OK?" class="Bool (strict)"("Value"=TRUE ("is OK?")) -> ()  [unwired: 2 in, 2 out]
                  }
                  event Value Change {
                    n193 = event-data() -> ()  [unwired: 1 in, 5 out]
                    n194 = property on="Array" class="Arr (strict)"() -> ("Value"=w185:refnum<vi>[])  [unwired: 2 in, 2 out]
                    n195 = for {
                      tunnel: w185 -> [w187] mode=indexing
                      n196 = control-ref of="Al bubbler"() -> (w186:refnum<vi>)
                      n197 = To More Specific Class(target class=w186, reference=w187) -> (specific class reference=w195:refnum<vi>)  [unwired: 1 in, 1 out]
                      n198 = property class="Clust (strict)"(reference=w195) -> ("Controls[]"=w194:refnum<vi>[])  [unwired: 1 in, 2 out]
                      n199 = control-ref of="Al Run"() -> (w188:refnum<vi>)
                      n200 = Index Array(array=w194, index=1) -> (element=w196:refnum<vi>)
                      n201 = Index Array(array=w194, index=2) -> (element=w192:refnum<vi>)
                      n202 = To More Specific Class(target class=w188, reference=w192) -> (specific class reference=w191:refnum<vi>, error out=w190:errorcluster)  [unwired: 1 in]
                      n203 = property class="Bool (strict)"(reference=w191, error in=w190) -> ("Value"=w189:bool)  [unwired: 2 out]
                      n204 = property class="Ctl"(reference=w196, "Visible"=w189) -> ()  [unwired: 1 in, 2 out]
                    }
                  }
                  event "Cancel": Value Change {
                    n205 = event-data() -> ()  [unwired: 1 in, 5 out]
                  }
                  event Value Change {
                    n206 = event-data() -> ()  [unwired: 1 in, 5 out]
                    n207 = control-ref of="Ga bubbler"() -> (w199:refnum<vi>)
                    n208 = call "dilutionCalcR.vi"("Clust Refnum"=w199) -> ()
                  }
                  event Value Change {
                    n209 = event-data() -> ()  [unwired: 1 in, 5 out]
                    n210 = control-ref of="Se bubbler"() -> (w200:refnum<vi>)
                    n211 = call "dilutionCalcR.vi"("Clust Refnum"=w200) -> ()
                  }
                }
              }
            }
            frame #2 {
              n212 = property on="is OK?" class="Bool (strict)"() -> ("Value"=w201:bool)  [unwired: 2 in, 2 out]
              n213 = Not(x=w201) -> (.not. x?=w205:bool)
              n214 = Current VI's Path() -> (path=w204:path)
              n215 = call "API_Edit.vi"("Cancel"=w205, "OK"=w201, "VI Path"=w204, "Argument List In"=w202) -> ("Argument List Out"=w203:string[])
            }
          }
          n216 = property class="VI"(reference=w112, "Front Panel.Open"=FALSE ("Front Panel Window:Open"), "FP.Behavior"=T5."Default" ("Front Panel Window:Behavior")) -> (reference out=w113:refnum<vi>)  [unwired: 1 in, 1 out]
          n217 = Close Reference(reference=w113) -> ()  [unwired: 1 in, 1 out]
        }
        frame "Start" {
          n218 = property on="prep_time" class="DigNum (strict)"() -> ("Value"=w210:dbl)  [unwired: 2 in, 2 out]
          n219 = Greater Than 0?(x=w210) -> (x > 0?=w209:bool)
          n220 = Not(x=w207) -> (.not. x?=w206:bool)
          n221 = And(x=w206, y=w209) -> (x .and. y?=w208:bool)
          n222 = case shown="True" w208 {
            frame False {
            }
            frame True {
              n223 = property on="Ga bubbler" class="Clust (strict)"() -> ("Value"=w220:T7)  [unwired: 2 in, 2 out]
              n224 = property on="P gas" class="Clust (strict)"() -> ("Value"=w218:T6)  [unwired: 2 in, 2 out]
              n225 = property on="Al bubbler" class="Clust (strict)"() -> ("Value"=w221:T6)  [unwired: 2 in, 2 out]
              n226 = property on="In bubbler" class="Clust (strict)"() -> ("Value"=w219:T6)  [unwired: 2 in, 2 out]
              n227 = property on="Se bubbler" class="Clust (strict)"() -> ("Value"=w215:T7)  [unwired: 2 in, 2 out]
              n228 = property on="As gas" class="Clust (strict)"() -> ("Value"=w217:T6)  [unwired: 2 in, 2 out]
              n229 = property on="P bubbler" class="Clust (strict)"() -> ("Value"=w216:T6)  [unwired: 2 in, 2 out]
              n230 = call "Set_V_III.vi"("Se bubbler"=w215, "P bubbler"=w216, "As gas"=w217, "P gas"=w218, "Run Started"=FALSE, "In bubbler"=w219, "Ga bubbler"=w220, "Al bubbler"=w221) -> ()  [unwired: 4 in]
            }
          }
          n231 = call "Set_Argument.vi"("Enable"=FALSE, "Argument"="run_started", "Argument List In"=w212) -> ("Argument List Out"=w211:string[])
        }
        frame "Run" {
          n232 = stacked-sequence {
            tunnel: w226 -> [_ w231 _ _]
            tunnel: w224 -> [w228 _ _ w305]
            tunnel: w225 -> [_ _ _ w303]
            tunnel: [_ _ _ w304] -> w223
            frame #0 {
              n233 = call "Get_Argument.vi"("Argument"="run_started", "Argument List"=w228) -> ("Enabled"=w227:bool)
              n234 = local write "run started"(w227) -> ()
            }
            frame #1 {
              n235 = property on="prep_time" class="DigNum (strict)"() -> ("Value"=w232:dbl)  [unwired: 2 in, 2 out]
              n236 = Greater Or Equal?(x=w231, y=w232) -> (x >= y?=w230:bool)
              n237 = local write "prep_done"(w230) -> ()
            }
            frame #2 {
              n238 = local read "run started"() -> (w234:bool)
              n239 = Not(x=w234) -> (.not. x?=w233:bool)
              n240 = stacked-sequence {
                tunnel: w233 -> [w236 w242 w251 w260 w269 w278 w287 w296]
                frame #0 {
                  n241 = case shown="True" w236 {
                    tunnel: ["run: " "pre-run: "] -> w235
                    frame False {
                    }
                    frame True {
                    }
                  }
                  n242 = property on="Status Out" class="Str"("Value"=w235) -> ()  [unwired: 2 in, 2 out]
                }
                frame #1 {
                  n243 = property on="Al bubbler" class="Clust (strict)"() -> ("Value"=w239:T6)  [unwired: 2 in, 2 out]
                  n244 = Unbundle By Name(w239) -> ("Run"=w241:bool, "Prep"=w240:bool)
                  n245 = property on="Status Out" class="Str"() -> ("Value"=w247:string)  [unwired: 2 in, 2 out]
                  n246 = call "flow_strings.vi"("string in"=w247, "is first in?"=TRUE, "name"="Al", "run source?"=w241, "prep source?"=w240, "is prep?"=w242) -> ("string out"=w246:string, "is first out?"=w245:bool)  [unwired: 1 in]
                  n247 = property on="Status Out" class="Str"("Value"=w246) -> ()  [unwired: 2 in, 2 out]
                  n248 = property on="first" class="Bool (strict)"("Value"=w245) -> ()  [unwired: 2 in, 2 out]
                }
                frame #2 {
                  n249 = property on="Ga bubbler" class="Clust (strict)"() -> ("Value"=w250:T7)  [unwired: 2 in, 2 out]
                  n250 = Unbundle By Name(w250) -> ("Bubbler (main).Run"=w249:bool, "Bubbler (main).Prep"=w248:bool)
                  n251 = property on="Status Out" class="Str"() -> ("Value"=w255:string)  [unwired: 2 in, 2 out]
                  n252 = property on="first" class="Bool (strict)"() -> ("Value"=w253:bool)  [unwired: 2 in, 2 out]
                  n253 = call "flow_strings.vi"("string in"=w255, "is first in?"=w253, "name"="Ga", "run source?"=w249, "prep source?"=w248, "is prep?"=w251) -> ("string out"=w256:string, "is first out?"=w252:bool)  [unwired: 1 in]
                  n254 = property on="Status Out" class="Str"("Value"=w256) -> ()  [unwired: 2 in, 2 out]
                  n255 = property on="first" class="Bool (strict)"("Value"=w252) -> ()  [unwired: 2 in, 2 out]
                }
                frame #3 {
                  n256 = property on="In bubbler" class="Clust (strict)"() -> ("Value"=w259:T6)  [unwired: 2 in, 2 out]
                  n257 = Unbundle By Name(w259) -> ("Run"=w258:bool, "Prep"=w257:bool)
                  n258 = property on="Status Out" class="Str"() -> ("Value"=w265:string)  [unwired: 2 in, 2 out]
                  n259 = property on="first" class="Bool (strict)"() -> ("Value"=w263:bool)  [unwired: 2 in, 2 out]
                  n260 = call "flow_strings.vi"("string in"=w265, "is first in?"=w263, "name"="In", "run source?"=w258, "prep source?"=w257, "is prep?"=w260) -> ("string out"=w262:string, "is first out?"=w261:bool)  [unwired: 1 in]
                  n261 = property on="Status Out" class="Str"("Value"=w262) -> ()  [unwired: 2 in, 2 out]
                  n262 = property on="first" class="Bool (strict)"("Value"=w261) -> ()  [unwired: 2 in, 2 out]
                }
                frame #4 {
                  n263 = property on="P gas" class="Clust (strict)"() -> ("Value"=w268:T6)  [unwired: 2 in, 2 out]
                  n264 = Unbundle By Name(w268) -> ("Run"=w267:bool, "Prep"=w266:bool)
                  n265 = property on="Status Out" class="Str"() -> ("Value"=w273:string)  [unwired: 2 in, 2 out]
                  n266 = property on="first" class="Bool (strict)"() -> ("Value"=w271:bool)  [unwired: 2 in, 2 out]
                  n267 = call "flow_strings.vi"("string in"=w273, "is first in?"=w271, "name"="PH3", "run source?"=w267, "prep source?"=w266, "is prep?"=w269) -> ("string out"=w272:string, "is first out?"=w270:bool)  [unwired: 1 in]
                  n268 = property on="Status Out" class="Str"("Value"=w272) -> ()  [unwired: 2 in, 2 out]
                  n269 = property on="first" class="Bool (strict)"("Value"=w270) -> ()  [unwired: 2 in, 2 out]
                }
                frame #5 {
                  n270 = property on="As gas" class="Clust (strict)"() -> ("Value"=w277:T6)  [unwired: 2 in, 2 out]
                  n271 = Unbundle By Name(w277) -> ("Run"=w276:bool, "Prep"=w275:bool)
                  n272 = property on="Status Out" class="Str"() -> ("Value"=w282:string)  [unwired: 2 in, 2 out]
                  n273 = property on="first" class="Bool (strict)"() -> ("Value"=w280:bool)  [unwired: 2 in, 2 out]
                  n274 = call "flow_strings.vi"("string in"=w282, "is first in?"=w280, "name"="AsH3", "run source?"=w276, "prep source?"=w275, "is prep?"=w278) -> ("string out"=w279:string, "is first out?"=w281:bool)  [unwired: 1 in]
                  n275 = property on="Status Out" class="Str"("Value"=w279) -> ()  [unwired: 2 in, 2 out]
                  n276 = property on="first" class="Bool (strict)"("Value"=w281) -> ()  [unwired: 2 in, 2 out]
                }
                frame #6 {
                  n277 = property on="P bubbler" class="Clust (strict)"() -> ("Value"=w286:T6)  [unwired: 2 in, 2 out]
                  n278 = Unbundle By Name(w286) -> ("Run"=w285:bool, "Prep"=w284:bool)
                  n279 = property on="Status Out" class="Str"() -> ("Value"=w292:string)  [unwired: 2 in, 2 out]
                  n280 = property on="first" class="Bool (strict)"() -> ("Value"=w290:bool)  [unwired: 2 in, 2 out]
                  n281 = call "flow_strings.vi"("string in"=w292, "is first in?"=w290, "name"="P liq", "run source?"=w285, "prep source?"=w284, "is prep?"=w287) -> ("string out"=w289:string, "is first out?"=w288:bool)  [unwired: 1 in]
                  n282 = property on="Status Out" class="Str"("Value"=w289) -> ()  [unwired: 2 in, 2 out]
                  n283 = property on="first" class="Bool (strict)"("Value"=w288) -> ()  [unwired: 2 in, 2 out]
                }
                frame #7 {
                  n284 = property on="Se bubbler" class="Clust (strict)"() -> ("Value"=w295:T7)  [unwired: 2 in, 2 out]
                  n285 = Unbundle By Name(w295) -> ("Bubbler (main).Run"=w294:bool, "Bubbler (main).Prep"=w293:bool)
                  n286 = property on="Status Out" class="Str"() -> ("Value"=w301:string)  [unwired: 2 in, 2 out]
                  n287 = property on="first" class="Bool (strict)"() -> ("Value"=w299:bool)  [unwired: 2 in, 2 out]
                  n288 = call "flow_strings.vi"("string in"=w301, "is first in?"=w299, "name"="Se", "run source?"=w294, "prep source?"=w293, "is prep?"=w296) -> ("string out"=w298:string, "is first out?"=w297:bool)  [unwired: 1 in]
                  n289 = property on="Status Out" class="Str"("Value"=w298) -> ()  [unwired: 2 in, 2 out]
                  n290 = property on="first" class="Bool (strict)"("Value"=w297) -> ()  [unwired: 2 in, 2 out]
                }
              }
            }
            frame #3 {
              n291 = property on="run started" class="Bool (strict)"() -> ("Value"=w307:bool)  [unwired: 2 in, 2 out]
              n292 = Not(x=w307) -> (.not. x?=w306:bool)
              n293 = property on="prep_done" class="Bool (strict)"() -> ("Value"=w308:bool)  [unwired: 2 in, 2 out]
              n294 = And(x=w308, y=w306) -> (x .and. y?=w302:bool)
              n295 = case shown="True" w302 {
                selector: w302 -> [_ w310]
                tunnel: w305 -> [w309 w313]
                tunnel: [w309 w312] -> w304
                tunnel: w303 -> [_ w311]
                frame False {
                }
                frame True {
                  n296 = stacked-sequence {
                    tunnel: w311 -> [w315 _]
                    tunnel: w313 -> [_ w325]
                    tunnel: [_ w324] -> w312
                    tunnel: w310 -> [w314 _]
                    frame #0 {
                      n297 = case shown="False" w315 {
                        tunnel: w314 -> [w323 _]
                        frame False {
                          n298 = property on="Ga bubbler" class="Clust (strict)"() -> ("Value"=w321:T7)  [unwired: 2 in, 2 out]
                          n299 = property on="In bubbler" class="Clust (strict)"() -> ("Value"=w320:T6)  [unwired: 2 in, 2 out]
                          n300 = property on="Se bubbler" class="Clust (strict)"() -> ("Value"=w316:T7)  [unwired: 2 in, 2 out]
                          n301 = property on="P gas" class="Clust (strict)"() -> ("Value"=w319:T6)  [unwired: 2 in, 2 out]
                          n302 = property on="Al bubbler" class="Clust (strict)"() -> ("Value"=w322:T6)  [unwired: 2 in, 2 out]
                          n303 = property on="As gas" class="Clust (strict)"() -> ("Value"=w318:T6)  [unwired: 2 in, 2 out]
                          n304 = property on="P bubbler" class="Clust (strict)"() -> ("Value"=w317:T6)  [unwired: 2 in, 2 out]
                          n305 = call "Set_V_III.vi"("Se bubbler"=w316, "P bubbler"=w317, "As gas"=w318, "P gas"=w319, "Run Started"=w323, "In bubbler"=w320, "Ga bubbler"=w321, "Al bubbler"=w322) -> ()  [unwired: 4 in]
                        }
                        frame True {
                        }
                      }
                    }
                    frame #1 {
                      n306 = call "Set_Argument.vi"("Enable"=TRUE, "Argument"="run_started", "Argument List In"=w325) -> ("Argument List Out"=w324:string[])
                    }
                  }
                }
              }
            }
          }
        }
        frame "End" {
        }
        frame "Idle" {
        }
      }
    }
  }
  "Argument List Out" <- w10
  n307 = control-ref of="Ga bubbler"() -> ()  [unwired: 1 out]
